vi "Command_Elevator.vi"(3 "Timeout":dbl=3.0, 4 "Allowable_Error":dbl=3.0, 5 "Set_Position":T1=enum."High_Rocket_Hatch_Panel_Floor", 6 "Startup":bool) -> (0 "Reinit":bool, 1 "Motor_Out":dbl, 2 "Completed":bool=TRUE)   [LabVIEW 2018]
uses:
  Subsytems/Elevator/Elevator_Enum_States.ctl
  Global_Variables/Sensor_Values.vi
  Global_Variables/Dashboard_Globals.vi
panel:
  in  "Max_Speed":dbl=1.0 format="%#_13g"
  in  "Gain_Down":dbl=5e-05
  in  "Gain_Up":dbl=0.0002
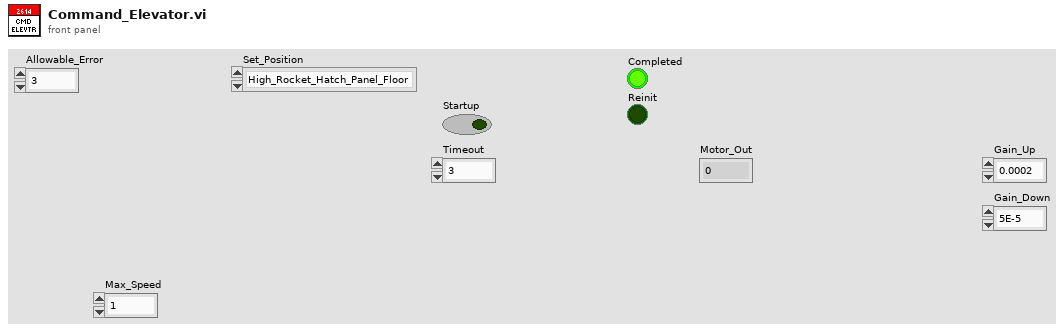
[diagram p1: front panel]
types:
  T1 = typedef "Elevator_Enum_States.ctl" = enum16{"Current_Position", "High_Rocket_Hatch_Panel_Floor", "High_Rocket_Hatch_Panel", "Mid_Rocket_Hatch_Panel_Floor", "Mid_Rocket_Hatch_Panel", "Low_Rocket_Hatch_Panel", "Cargo_Ship_Hatch_Panel", "Loading_Station_Hatch_Panel", "Ground_Pickup_Hatch_Panel", "High_Rocket_Cargo", "Mid_Rocket_Cargo", "Low_Rocket_Cargo", "Cargo_Ship_Cargo", "Loading_Station_Cargo", "Ground_Pickup_Cargo", "Depot_Pickup_Cargo", "Stow_Cargo"}
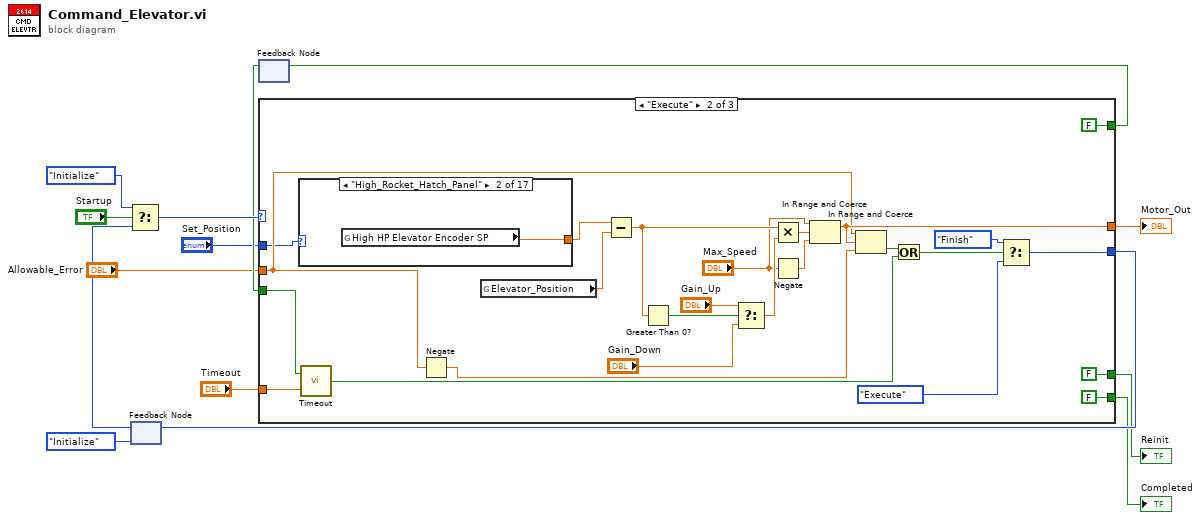
[diagram p0: block diagram]
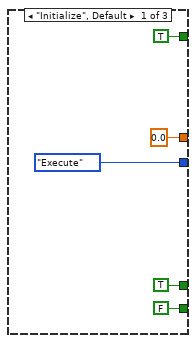
[diagram p2: hidden frame]
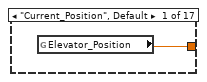
[diagram p3: hidden frame]
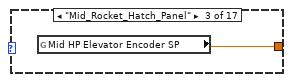
[diagram p4: hidden frame]
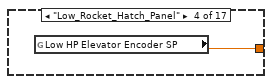
[diagram p5: hidden frame]
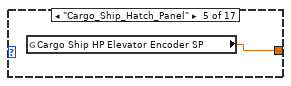
[diagram p6: hidden frame]
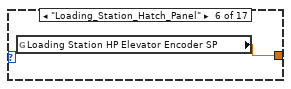
[diagram p7: hidden frame]
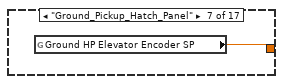
[diagram p8: hidden frame]
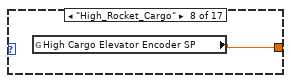
[diagram p9: hidden frame]
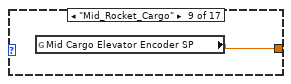
[diagram p10: hidden frame]
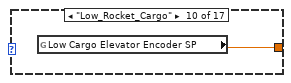
[diagram p11: hidden frame]
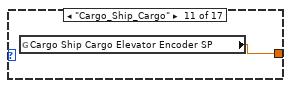
[diagram p12: hidden frame]
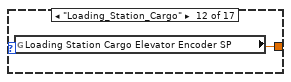
[diagram p13: hidden frame]
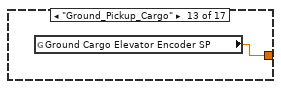
[diagram p14: hidden frame]
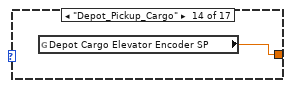
[diagram p15: hidden frame]
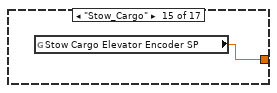
[diagram p16: hidden frame]
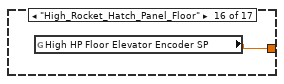
[diagram p17: hidden frame]
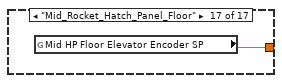
[diagram p18: hidden frame]
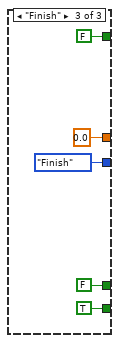
[diagram p19: hidden frame]
diagram:
  n1 = feedback #1(enum16{"Initialize", "Execute", "Finish"}."Initialize" ("f")) -> (w10:enum16{"Initialize", "Execute", "Finish"})
  n2 = Select(t=enum16{"Initialize", "Execute", "Finish"}."Initialize", s="Startup", f=w10) -> (s? t:f=w14:enum16{"Initialize", "Execute", "Finish"})
  n3 = feedback #2() -> (w8:bool)  [unwired: 1 in]
  n4 = case shown="\"Execute\"" w14 {
    tunnel: [enum16{"Initialize", "Execute", "Finish"}."Execute" w41 enum16{"Initialize", "Execute", "Finish"}."Finish" ("f")] -> w11
    tunnel: w8 -> [_ w39 _]
    tunnel: [TRUE FALSE FALSE] -> w9
    tunnel: [FALSE FALSE TRUE] -> w7
    tunnel: [TRUE FALSE FALSE] -> w6
    tunnel: "Timeout" -> [_ w36 _]
    tunnel: [0.0 w25 0.0] -> w3
    tunnel: "Set_Position" -> [_ w21 _]
    tunnel: "Allowable_Error" -> [_ w22 _]
    frame "Initialize", Default {
    }
    frame "Execute" {
      n5 = case shown="\"High_Rocket_Hatch_Panel\"" w21 {
        tunnel: [w45 w46 w47 w48 w49 w50 w51 w52 w53 w54 w55 w56 w57 w58 w59 w60 w61] -> w20
        frame "Current_Position", Default {
          n6 = global read "Sensor_Values.vi" "Elevator_Position"() -> (w45:dbl)
        }
        frame "High_Rocket_Hatch_Panel" {
          n7 = global read "Dashboard_Globals.vi" "High HP Elevator Encoder SP"() -> (w46:dbl)
        }
        frame "Mid_Rocket_Hatch_Panel" {
          n8 = global read "Dashboard_Globals.vi" "Mid HP Elevator Encoder SP"() -> (w47:dbl)
        }
        frame "Low_Rocket_Hatch_Panel" {
          n9 = global read "Dashboard_Globals.vi" "Low HP Elevator Encoder SP"() -> (w48:dbl)
        }
        frame "Cargo_Ship_Hatch_Panel" {
          n10 = global read "Dashboard_Globals.vi" "Cargo Ship HP Elevator Encoder SP"() -> (w49:dbl)
        }
        frame "Loading_Station_Hatch_Panel" {
          n11 = global read "Dashboard_Globals.vi" "Loading Station HP Elevator Encoder SP"() -> (w50:dbl)
        }
        frame "Ground_Pickup_Hatch_Panel" {
          n12 = global read "Dashboard_Globals.vi" "Ground HP Elevator Encoder SP"() -> (w51:dbl)
        }
        frame "High_Rocket_Cargo" {
          n13 = global read "Dashboard_Globals.vi" "High Cargo Elevator Encoder SP"() -> (w52:dbl)
        }
        frame "Mid_Rocket_Cargo" {
          n14 = global read "Dashboard_Globals.vi" "Mid Cargo Elevator Encoder SP"() -> (w53:dbl)
        }
        frame "Low_Rocket_Cargo" {
          n15 = global read "Dashboard_Globals.vi" "Low Cargo Elevator Encoder SP"() -> (w54:dbl)
        }
        frame "Cargo_Ship_Cargo" {
          n16 = global read "Dashboard_Globals.vi" "Cargo Ship Cargo Elevator Encoder SP"() -> (w55:dbl)
        }
        frame "Loading_Station_Cargo" {
          n17 = global read "Dashboard_Globals.vi" "Loading Station Cargo Elevator Encoder SP"() -> (w56:dbl)
        }
        frame "Ground_Pickup_Cargo" {
          n18 = global read "Dashboard_Globals.vi" "Ground Cargo Elevator Encoder SP"() -> (w57:dbl)
        }
        frame "Depot_Pickup_Cargo" {
          n19 = global read "Dashboard_Globals.vi" "Depot Cargo Elevator Encoder SP"() -> (w58:dbl)
        }
        frame "Stow_Cargo" {
          n20 = global read "Dashboard_Globals.vi" "Stow Cargo Elevator Encoder SP"() -> (w59:dbl)
        }
        frame "High_Rocket_Hatch_Panel_Floor" {
          n21 = global read "Dashboard_Globals.vi" "High HP Floor Elevator Encoder SP"() -> (w60:dbl)
        }
        frame "Mid_Rocket_Hatch_Panel_Floor" {
          n22 = global read "Dashboard_Globals.vi" "Mid HP Floor Elevator Encoder SP"() -> (w61:dbl)
        }
      }
      n23 = call "Timeout.vi"("Timeout"=w36, "Initialize"=w39) -> ("Timed Out?"=w37:bool)
      n24 = Negate(x=w22) -> (-x=w24:dbl)
      n25 = global read "Sensor_Values.vi" "Elevator_Position"() -> (w26:dbl)
      n26 = Subtract(x=w20, y=w26) -> (x-y=w33:dbl)
      n27 = Greater Than 0?(x=w33) -> (x > 0?=w34:bool)
      n28 = Select(t="Gain_Up", s=w34, f="Gain_Down") -> (s? t:f=w30:dbl)
      n29 = Multiply(x=w33, y=w30) -> (x*y=w29:dbl)
      n30 = Negate(x="Max_Speed") -> (-x=w27:dbl)
      n31 = In Range and Coerce(upper limit="Max_Speed", x=w29, lower limit=w27) -> (coerced(x)=w25:dbl)  [unwired: 1 out]
      n32 = In Range and Coerce(upper limit=w22, x=w25, lower limit=w24) -> (In Range?=w23:bool)  [unwired: 1 out]
      n33 = Or(x=w23, y=w37) -> (x .or. y?=w35:bool)
      n34 = Select(t=enum16{"Initialize", "Execute", "Finish"}."Finish", s=w35, f=enum16{"Initialize", "Execute", "Finish"}."Execute") -> (s? t:f=w41:enum16{"Initialize", "Execute", "Finish"})
    }
    frame "Finish" {
    }
  }
  "Completed" <- w7
  "Reinit" <- w6
  "Motor_Out" <- w3
  n35 = feedback-in #1(w11) -> ()
  n36 = feedback-in #2(w9) -> ()
